vi "forceOutputState.vi"(8 "error in (no error)":errorcluster, 9 "calibratedValues":dbl[](array[numeric]), 10 "channel_addresses":string[](array[string]), 11 "K2602 in":refnum<class "K2602.lvclass">) -> (0 "error out":errorcluster, 3 "K2602 out":refnum<class "K2602.lvclass">)   [LabVIEW 2011, in "Hardware.lvlib" / "Channels.lvlib" / "K2602.lvclass"]
uses:
  K2602.lvclass
  AnalogOutput.lvclass
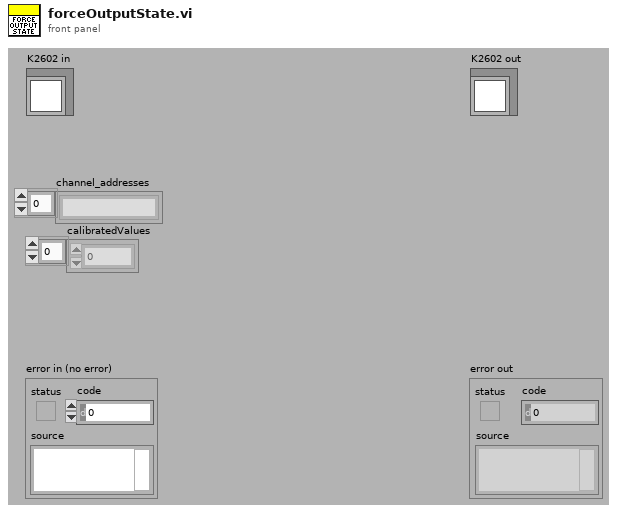
[diagram p1: front panel]
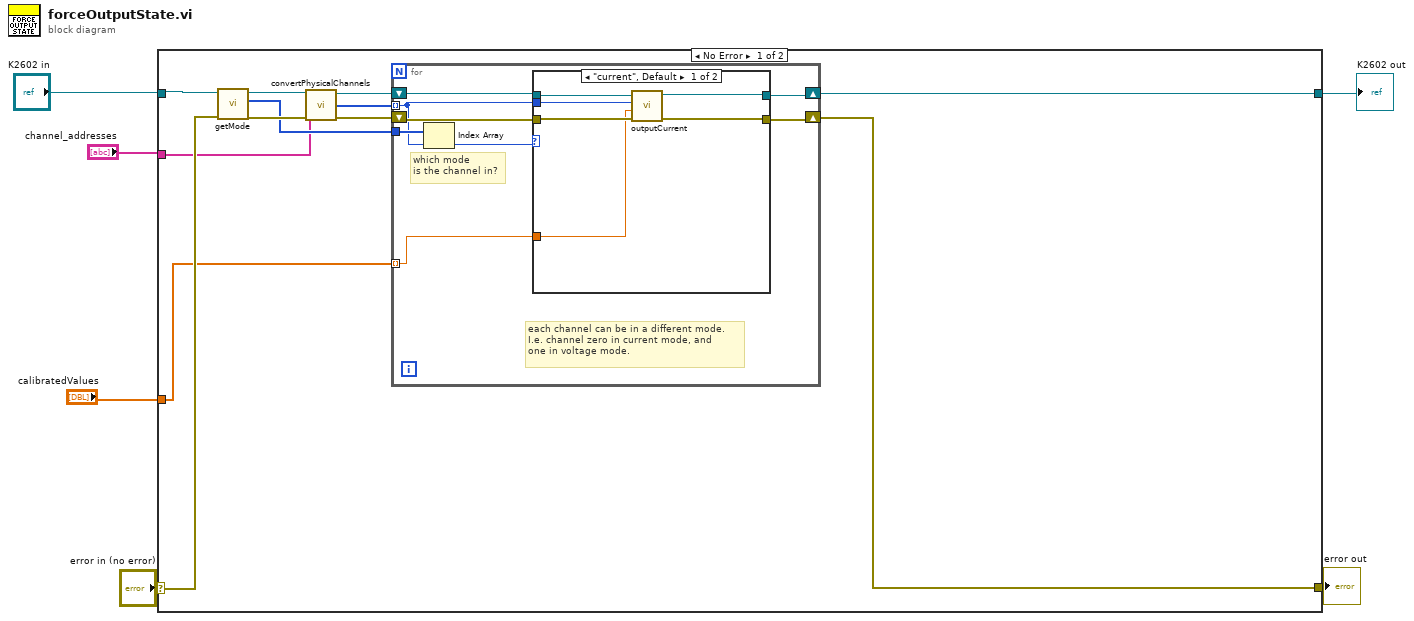
[diagram p0: block diagram]
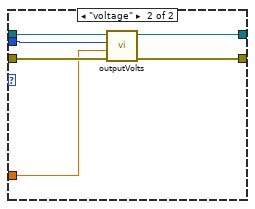
[diagram p2: hidden frame]
diagram:
  n1 = case shown="No Error" "error in (no error)" {
    selector: "error in (no error)" -> [w17 w40]
    tunnel: [w14 w39] -> w1
    tunnel: "K2602 in" -> [w18 w39]
    tunnel: [w8 w40] -> w2
    tunnel: "calibratedValues" -> [w9 _]
    tunnel: "channel_addresses" -> [w7 _]
    frame No Error {
      n2 = call "getMode.vi"("error in (no error)"=w17, "AnalogOutput in"=w18) -> ("error out"=w15:errorcluster, "mode"=w11:enum16{"current", "voltage"}[], "AnalogOutput out"=w16:refnum<class "K2602.lvclass">)  [unwired: 7 in]
      n3 = call "convertPhysicalChannels.vi"("error in (no error)"=w15, "physicalChannels"=w7, "K2602 in"=w16) -> ("error out"=w10:errorcluster, "channel"=w12:i32[], "K2602 out"=w13:refnum<class "K2602.lvclass">)  [unwired: 6 in]
      n4 = for {
        shift-right: [w23] -> w14
        shift-left: w13 -> [w24]
        tunnel: w12 -> [w19] mode=indexing
        tunnel: w11 -> [w26]
        tunnel: w9 -> [w20] mode=indexing
        shift-right: [w21] -> w8
        shift-left: w10 -> [w22]
        # "each channel can be in a different mode.\nI.e. channel zero in current mode, and \none in voltage mode."
        # "which mode\nis the channel in?"
        n5 = Index Array(array=w26, index=w19) -> (element=w25:enum16{"current", "voltage"})
        n6 = case shown="\"current\", Default" w25 {
          tunnel: w24 -> [w32 w38]
          tunnel: [w27 w37] -> w23
          tunnel: w22 -> [w31 w36]
          tunnel: [w30 w35] -> w21
          tunnel: w20 -> [w28 w33]
          tunnel: w19 -> [w29 w34]
          frame "current", Default {
            n7 = call "outputCurrent.vi"("error in (no error)"=w31, "calibratedValue"=w28, "channel"=w29, "K2602 in"=w32) -> ("error out"=w30:errorcluster, "K2602 out"=w27:refnum<class "K2602.lvclass">)  [unwired: 6 in]
          }
          frame "voltage" {
            n8 = call "outputVolts.vi"("error in (no error)"=w36, "calibratedValue"=w33, "channel"=w34, "K2602 in"=w38) -> ("error out"=w35:errorcluster, "K2602 out"=w37:refnum<class "K2602.lvclass">)  [unwired: 6 in]
          }
        }
      }
    }
    frame Error {
    }
  }
  "error out" <- w2
  "K2602 out" <- w1
